vi "Fetch Waveform.vi"(8 "error in (no error)":errorcluster {"code" format="%.0x"}, 10 "Channel Name (\"Channel 1\")":string(combo)="CHAN1", 11 "VISA Resource Name":refnum<visa-resource-name>) -> (0 "error out":errorcluster {"code" format="%.0x"}, 1 "x increment":dbl caption="x Increment" format="%^.2e", 2 "initial x":dbl caption="Initial x" format="%^.2e", 3 "VISA Resource Name Out":refnum<visa-resource-name>, 4 "waveform array":dbl[](array[numeric]) caption="Waveform Array" format="%.2f", 5 "actual points":u32 caption="Actual Points")   [LabVIEW 2011, in "Agilent 546XX Series.lvlib"]
doc: "This VI returns the waveform the oscilloscope acquires for the channel you specify. The waveform is from an acquisition that you previously initiated. \n\nYou use the ag546xx Initiate Acquisition VI to start an acquisition on the channels that you enable with the ag546xx Configure Channel VI. The oscilloscope acquires waveforms for the enabled channels concurrently. You must call this VI separately for each enabled channel to obtain the waveforms.\n\nYou can call the ag546xx Read Waveform VI instead of the ag546xx Initiate Acquisition VI. The ag546xx Read Waveform VI starts an acquisition on all enabled channels, waits for the acquisition to complete, and returns the waveform for the channel you specify. You call this VI to obtain the waveforms for each of the remaining channels.\n\nNotes:\n\n(1) After this VI executes, each element in the Waveform Array is either a voltage or a value indicating that the oscilloscope could not sample a voltage.\n\n(2) This VI does not check the instrument status. Typically, you call this VI only in a sequence of calls to other low-level driver VIs. The sequence performs one operation. You use the low-level VIs to optimize one or more aspects of interaction with the instrument. If you want to check the instrument status, call the ag546xx Error-Query VI at the conclusion of the sequence."
uses:
  Agilent 546XX Series.lvlib
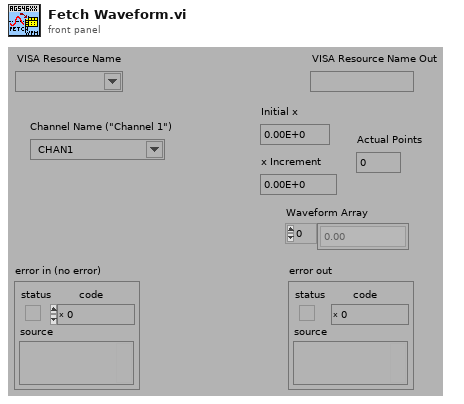
[diagram p1: front panel]
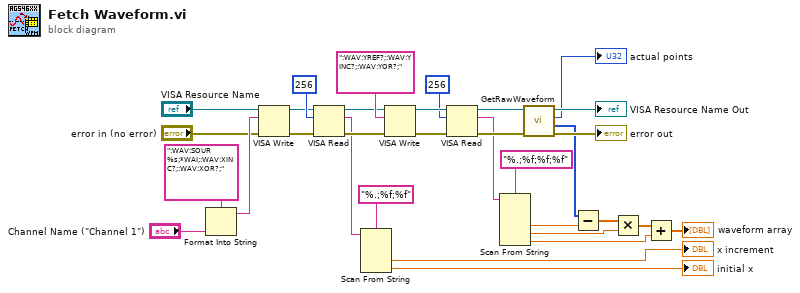
[diagram p0: block diagram]
diagram:
  n1 = Format Into String(format string=":WAV:SOUR %s;*WAI;:WAV:XINC?;:WAV:XOR?;", "Channel Name (\"Channel 1\")") -> (resulting string=w31:string)  [unwired: 2 in, 1 out]
  n2 = VISA Write(VISA resource name="VISA Resource Name", write buffer=w31, error in (no error)="error in (no error)") -> (VISA resource name out=w8:refnum<visa-resource-name>, error out=w7:errorcluster)  [unwired: 1 out]
  n3 = VISA Read(VISA resource name=w8, byte count=u32 256, error in (no error)=w7) -> (VISA resource name out=w6:refnum<visa-resource-name>, read buffer=w4:string, error out=w5:errorcluster)  [unwired: 1 out]
  n4 = Scan From String(format string="%.;%f;%f", input string=w4) -> (output 1=→"x increment":dbl, output 2=→"initial x":dbl)  [unwired: 4 in, 3 out]
  n5 = VISA Write(VISA resource name=w6, write buffer=":WAV:YREF?;:WAV:YINC?;:WAV:YOR?;", error in (no error)=w5) -> (VISA resource name out=w30:refnum<visa-resource-name>, error out=w29:errorcluster)  [unwired: 1 out]
  n6 = VISA Read(VISA resource name=w30, byte count=u32 256, error in (no error)=w29) -> (VISA resource name out=w28:refnum<visa-resource-name>, read buffer=w22:string, error out=w27:errorcluster)  [unwired: 1 out]
  n7 = Scan From String(format string="%.;%f;%f;%f", input string=w22) -> (output 1=w20:dbl, output 2=w18:dbl, output 3=w16:dbl)  [unwired: 5 in, 3 out]
  n8 = call "GetRawWaveform.vi"("error in"=w27, "VISA Resource Name"=w28) -> ("error out"=→"error out":errorcluster, "Waveform Array"=w14:u32[], "Number of Points"=→"actual points":u32, "VISA Resource Name Out"=→"VISA Resource Name Out":refnum<visa-resource-name>)  [unwired: 5 in, 1 out]
  n9 = Subtract(x=w14, y=w20) -> (x-y=w19:dbl[])
  n10 = Multiply(x=w19, y=w18) -> (x*y=w17:dbl[])
  n11 = Add(x=w17, y=w16) -> (x+y=→"waveform array":dbl[])
